vi "Load Config.vi"(6 "Constants":refnum<class "Sequence Constants.lvclass">, 8 "error in (no error)":refnum<class "MultiErrors.lvclass">, 10 "Config Element":refnum<class "Config Element.lvclass">, 11 "Time Condition Config in":refnum<class "Time Condition Config.lvclass">) -> (0 "error out":refnum<class "MultiErrors.lvclass">, 3 "Time Condition Config out":refnum<class "Time Condition Config.lvclass">)   [LabVIEW 2020, in "VolatusSeqConfig.lvlib" / "Time Condition Config.lvclass"]
uses:
  Time Condition Config.lvclass
  VolatusErrorUtilities/MultiErrors/MultiErrors.lvclass
  lv-cdm/CDM-Config/Config Element/Config Element.lvclass
  Sequence Constants/Sequence Constants.lvclass
  Timer.ctl
  Time Condition Config.lvclass/Time Condition Config.ctl
  VolatusSeqConfig.lvlib
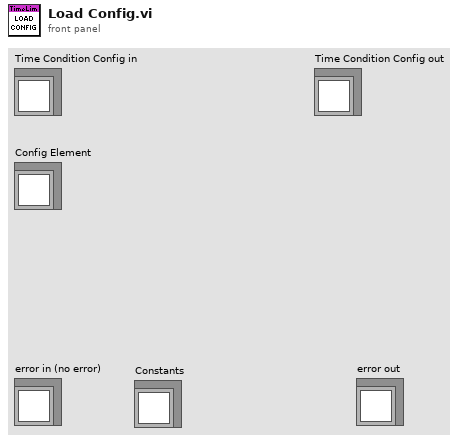
[diagram p1: front panel]
types:
  T1 = typedef "VolatusSeqConfig.lvlib/Timer.ctl" = enum16{"Sequence", "State", "Wall"}
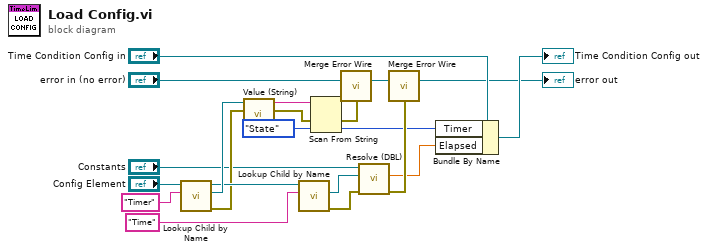
[diagram p0: block diagram]
diagram:
  n1 = call "Lookup Child by Name.vi"("Name"="Timer", "Config Element in"="Config Element") -> ("error out"=w7:errorcluster, "Child"=w16:refnum<class "Config Element.lvclass">, "Config Element out"=w11:refnum<class "Config Element.lvclass">)  [unwired: 6 in, 1 out]
  n2 = call "Value (String).vi"("error in (no error)"=w7, "Config Element in"=w16) -> ("error out"=w6:errorcluster, "String Value"=w15:string)  [unwired: 8 in]
  n3 = call "Lookup Child by Name.vi"("Name"="Time", "Config Element in"=w11) -> ("error out"=w5:errorcluster, "Child"=w9:refnum<class "Config Element.lvclass">)  [unwired: 6 in, 2 out]
  n4 = Scan From String(input string=w15, error in=w6, default 1=Timer."State" ("Timer")) -> (error out=w3:errorcluster, output 1=w12:T1)  [unwired: 2 in, 2 out]
  n5 = call "Merge Error Wire.vi"("error in (no error)"=w3, "MultiErrors in"="error in (no error)") -> ("MultiErrors out"=w4:refnum<class "MultiErrors.lvclass">)  [unwired: 13 in]
  n6 = call "Resolve (DBL).vi"("error in (no error)"=w5, "Element"=w9, "Sequence Constants in"="Constants") -> ("error out"=w21:errorcluster, "DBL Value"=w8:dbl)  [unwired: 6 in, 1 out]
  n7 = call "Merge Error Wire.vi"("error in (no error)"=w21, "MultiErrors in"=w4) -> ("MultiErrors out"=→"error out":refnum<class "MultiErrors.lvclass">)  [unwired: 13 in]
  n8 = Bundle By Name(cluster="Time Condition Config in", "Timer"=w12, "Elapsed"=w8) -> (→"Time Condition Config out":refnum<class "Time Condition Config.lvclass">)
